vi "GOMDBTS2048 spectral Get Counts Pixel.vi"(8 "error in (no error)":errorcluster, 11 "handle":i32) -> (0 "error out":errorcluster, 2 "function return":i32, 3 "counts":dbl[](array[numeric]))   [LabVIEW 2015, in "GOMDBTS2048.lvlib"]
doc: "GOBTS2048DLL int __stdcall GOMDBTS2048_spectralGetCountsPixel(int handle, double* counts);"
uses:
  GOMDBTS2048.lvlib
  runtime/GOMDBTS2048.dll
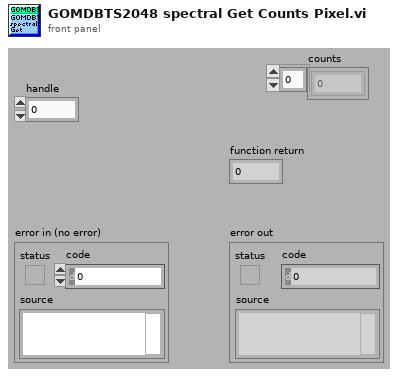
[diagram p1: front panel]
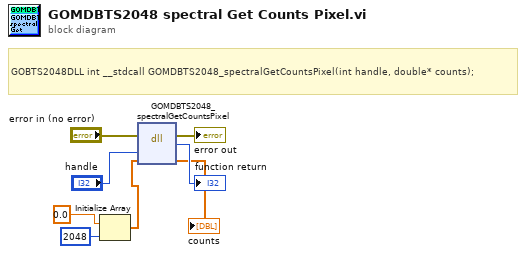
[diagram p0: block diagram]
diagram:
  # "GOBTS2048DLL int __stdcall GOMDBTS2048_spectralGetCountsPixel(int handle, double* counts);"
  n1 = Initialize Array(0.0 ("element"), 2048 ("dimension size")) -> (w1:dbl[])
  n2 = dll-call lib="C:/Users/rkoch/Documents/GO_Library/runtime/GOMDBTS2048.*" fn="GOMDBTS2048_spectralGetCountsPixel"(error in="error in (no error)", "handle"="handle", "counts"=w1) -> (error out=→"error out":errorcluster, "return type"=→"function return":i32, "counts"=→"counts":dbl[])  [unwired: 3 in, 1 out]
